vi "Clamp Max.vi"() -> ()   [LabVIEW 2014]
doc: "This example demonstrates the capabilities of the Max Clamp algorithm on a test image. You can also use this example to experiment using your own images and settings."
uses:
  <vilib>/vision/NI_Vision_Development_Module.lvlib
panel:
  in  "Clamp Settings":T1={"Angle Range (+/-)"=5.0, "Edge Polarity"={"Start"=0, "End"=0}} {"Edge Polarity"."End" items=["Any", "Rising", "Falling"]; "Edge Polarity"."Start" items=["Any", "Rising", "Falling"]}
  out "Clamp Results":T2 {"Angle (Relative)" format="%.3f"; "Angle (Absolute)" format="%.3f"; "Distance (Real World)" format="%.3f"; "Distance (Pixels)" format="%.3f"}
  in  "Curve Extraction Settings":T3={"Extraction Mode"=0, "Edge Threshold"=40, "Edge Filter Size"=1, "Min Length"=15, "Row Search Step Size"=10, "Col Search Step Size"=10, "Max Endpoint Gap"=5, "Closed"=FALSE, "Subpixel"=FALSE} {"Max Endpoint Gap" min=0; "Col Search Step Size" min=1 max=255 step=1; "Row Search Step Size" min=1 max=255 step=1; "Min Length" min=0; "Edge Filter Size" items=["Fine", "Normal", "Contour Tracing"]; "Edge Threshold" min=1 max=350 step=1; "Extraction Mode" items=["Normal", "Uniform Regions"]}
  out "Image":T4(plugin-control)
  in  "Stop":bool
  # "Overview: Demonstrates how to use the IMAQ Clamp Max function to find the maximum distance between the curves of an object.\nRequirements: Vision Development Software.\nInstructions:\n1. Run the VI.\n2. Draw a Region of Interest in the image or change the Curve Extraction Settings or Clamp Settings to see how the Max Clamp function works."
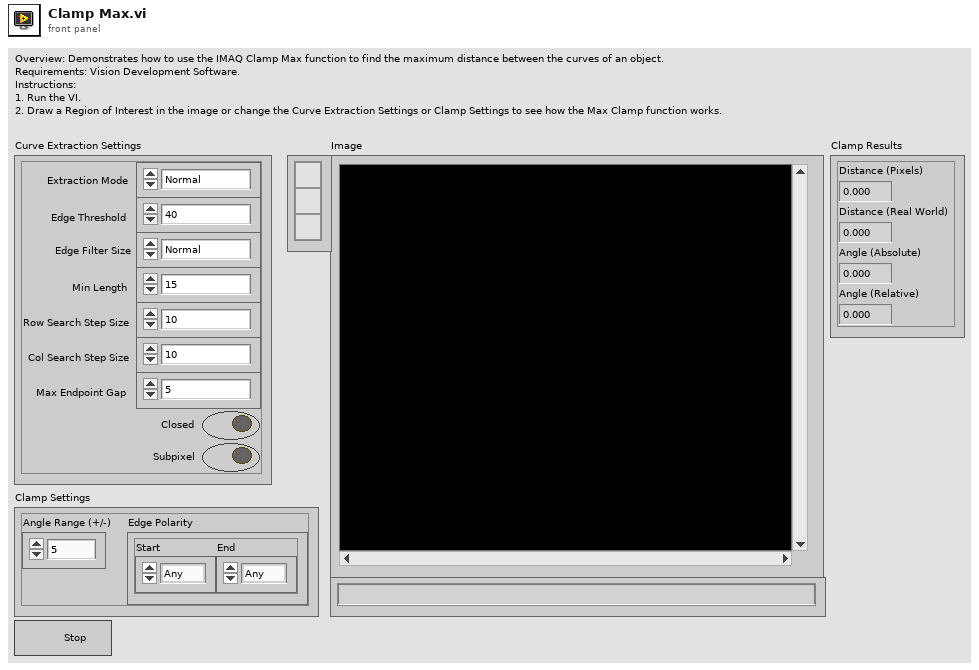
[diagram p1: front panel]
types:
  T1 = cluster{"Angle Range (+/-)":dbl, "Edge Polarity":cluster{"Start":u32, "End":u32}}
  T2 = cluster{"Distance (Pixels)":dbl, "Distance (Real World)":dbl, "Angle (Absolute)":dbl, "Angle (Relative)":dbl}
  T3 = cluster{"Extraction Mode":u32, "Edge Threshold":i32, "Edge Filter Size":u32, "Min Length":i32, "Row Search Step Size":i32, "Col Search Step Size":i32, "Max Endpoint Gap":i32, "Closed":bool, "Subpixel":bool}
  T4 = typedef "IMAQ Image.ctl" = refnum<image>
  T5 = typedef "ROI Descriptor" = cluster{"Global Rectangle":i32[], "Contours":cluster{"ID":enum32{"External", "Internal"}, "Type":u32, "Coordinates":i32[]}[]}
  T6 = typedef "Image Type" = u32
  T7 = cluster{"Show Search Area":bool, "Show Curves":bool, "Show Clamp Locations":bool, "Show Result":bool, "Search Area Color":u32, "Curves Color":u32, "Clamp Locations Color":u32, "Result Color":u32, "Overlay Group Name":string}
  T8 = cluster{"Global Rectangle":i32[], "Contours":cluster{"Contour Type":u32, "ROI Type":u32, "Points":i32[]}[]}
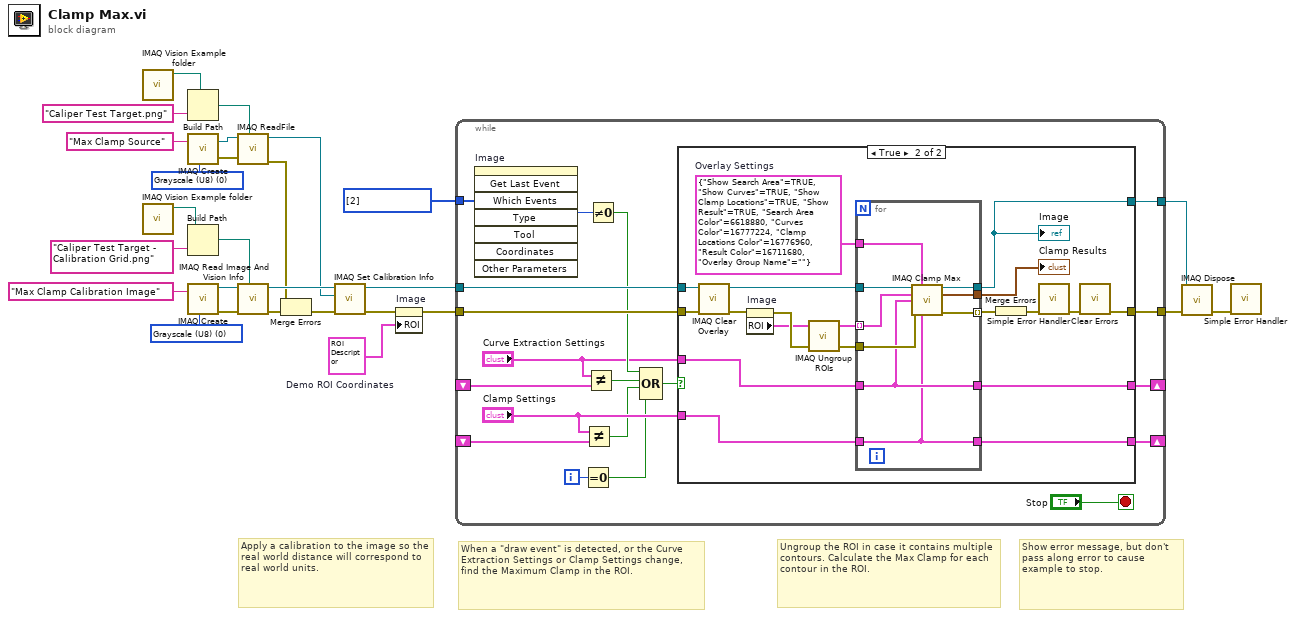
[diagram p0: block diagram]
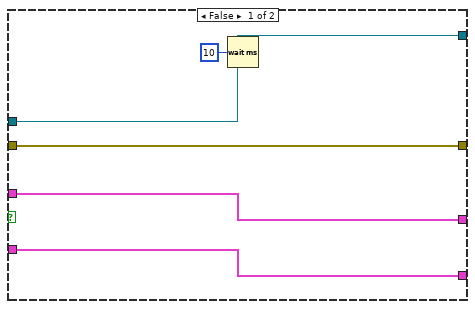
[diagram p2: hidden frame]
diagram:
  w8 = T5 {"Global Rectangle"=[94, 43, 1305, 1017], "Contours"=[{"ID"=enum."External", "Type"=12, "Coordinates"=[94, 214, 224, 312, 0]}, {"ID"=enum."External", "Type"=12, "Coordinates"=[232, 213, 372, 311, 321805]}, {"ID"=enum."External", "Type"=12, "Coordinates"=[143, 362, 220, 410, 0]}, {"ID"=enum."External", "Type"=12, "Coordinates"=[102, 475, 219, 529, 0]}, {"ID"=enum."External", "Type"=12, "Coordinates"=[226, 467, 369, 539, 315305]}, {"ID"=enum."External", "Type"=12, "Coordinates"=[221, 635, 380, 786, 359893]}, {"ID"=enum."External", "Type"=12, "Coordinates"=[538, 44, 687, 107, 359893]}, {"ID"=enum."External", "Type"=12, "Coordinates"=[501, 185, 671, 254, 359893]}, {"ID"=enum."External", "Type"=12, "Coordinates"=[501, 599, 671, 661, 359893]}, {"ID"=enum."External", "Type"=12, "Coordinates"=[729, 602, 899, 664, 314592]}, {"ID"=enum."External", "Type"=12, "Coordinates"=[491, 770, 679, 826, 0]}, {"ID"=enum."External", "Type"=12, "Coordinates"=[738, 781, 898, 817, 0]}, {"ID"=enum."External", "Type"=12, "Coordinates"=[498, 954, 669, 972, 0]}, {"ID"=enum."External", "Type"=12, "Coordinates"=[741, 949, 890, 974, 322432]}, {"ID"=enum."External", "Type"=12, "Coordinates"=[999, 450, 1293, 565, 0]}, {"ID"=enum."External", "Type"=12, "Coordinates"=[983, 106, 1305, 217, 0]}, {"ID"=enum."External", "Type"=12, "Coordinates"=[1152, 132, 1301, 191, 0]}, {"ID"=enum."External", "Type"=12, "Coordinates"=[961, 755, 1143, 952, 0]}, {"ID"=enum."External", "Type"=12, "Coordinates"=[233, 851, 379, 1005, 0]}]}  # Demo ROI Coordinates
  w12 = i32[] [2] items=["No Event"=0, "Click Event"=1, "Draw Event"=2, "Size Event"=4, "Scroll Event"=5, "Double Click Event"=8] ("Which Events")
  w26 = T6 0 items=["Grayscale (U8)", "Grayscale (I16)", "Grayscale (SGL)", "Complex (CSG)", "RGB (U32)", "HSL (U32)", "RGB (U64)", "Grayscale (U16)"] ("Image Type")
  w27 = T6 0 items=["Grayscale (U8)", "Grayscale (I16)", "Grayscale (SGL)", "Complex (CSG)", "RGB (U32)", "HSL (U32)", "RGB (U64)", "Grayscale (U16)"] ("Image Type")
  # "Show error message, but don't pass along error to cause example to stop."
  # "Ungroup the ROI in case it contains multiple contours. Calculate the Max Clamp for each contour in the ROI."
  # "When a \"draw event\" is detected, or the Curve Extraction Settings or Clamp Settings change, find the Maximum Clamp in the ROI."
  # "Apply a calibration to the image so the real world distance will correspond to real world units."
  n1 = call "IMAQ Vision Example folder.vi"() -> ("Example Image Path"=w16:path)  [unwired: 11 in]
  n2 = call "IMAQ Vision Example folder.vi"() -> ("Example Image Path"=w22:path)  [unwired: 11 in]
  n3 = Build Path(base path=w16, name or relative path="Caliper Test Target.png") -> (appended path=w15:path)
  n4 = call "IMAQ Create"("Image Name"="Max Clamp Source", "Image Type"=w27) -> ("New Image"=w18:T4, "error out"=w4:errorcluster)  [unwired: 2 in, 1 out]
  n5 = Build Path(base path=w22, name or relative path="Caliper Test Target - Calibration Grid.png") -> (appended path=w20:path)
  n6 = call "IMAQ Create"("Image Name"="Max Clamp Calibration Image", "Image Type"=w26) -> ("New Image"=w21:T4, "error out"=w5:errorcluster)  [unwired: 2 in, 1 out]
  n7 = call "IMAQ ReadFile"("File Path"=w15, "error in (no error)"=w4, "Image"=w18) -> ("error out"=w3:errorcluster, "Image Out"=w14:T4)  [unwired: 2 in, 5 out]
  n8 = call "IMAQ Read Image And Vision Info"("File Path"=w20, "error in (no error)"=w5, "Image"=w21) -> ("error out"=w2:errorcluster, "Image Out"=w19:T4)  [unwired: 1 in, 6 out]
  n9 = Merge Errors(w3, w2) -> (w1:errorcluster)
  n10 = call "IMAQ Set Calibration Info"("error in (no error)"=w1, "Image Dst"=w14, "Image Src"=w19) -> ("error out"=w7:errorcluster, "Calibrated Image"=w13:T4)  [unwired: 1 in, 6 out]
  n11 = property on="Image" class="ImageControl"(error in=w7, "ROI"=w8) -> (error out=w6:errorcluster)  [unwired: 1 in, 1 out]
  n12 = while {
    tunnel: w13 -> [w42]
    tunnel: w6 -> [w43]
    tunnel: w12 -> [w45]
    tunnel: [w29] -> w10
    tunnel: [w28] -> w11
    shift-right: [w31] -> _
    shift-left: _ -> [w41]
    shift-right: [w30] -> _
    shift-left: _ -> [w39]
    i -> [w46]
    stop <- "Stop" stop-if-true
    n13 = invoke on="Image" class="ImageControl" method="Get Last Event"("Which Events"=w45) -> ("Type"=w35:i32)  [unwired: 7 in, 7 out]
    n14 = Equal To 0?(x=w46) -> (x = 0?=w36:bool)
    n15 = Not Equal?(x="Clamp Settings", y=w41) -> (x != y?=w37:bool)
    n16 = Not Equal?(x="Curve Extraction Settings", y=w39) -> (x != y?=w38:bool)
    n17 = Not Equal To 0?(x=w35) -> (x != 0?=w34:bool)
    n18 = Compound Arithmetic op=OR(w34, w38, w37, w36) -> (w33:bool)
    n19 = case shown="True" w33 {
      tunnel: w42 -> [w47 w70]
      tunnel: w43 -> [w48 w69]
      tunnel: "Clamp Settings" -> [w50 w52]
      tunnel: "Curve Extraction Settings" -> [w49 w62]
      tunnel: [w50 w56] -> w31
      tunnel: [w49 w57] -> w30
      tunnel: [w48 w54] -> w29
      tunnel: [w47 w53] -> w28
      frame False {
        n20 = Wait (ms)(milliseconds to wait=u32 10) -> ()  [unwired: 1 out]
      }
      frame True {
        w61 = T7 {"Show Search Area"=TRUE, "Show Curves"=TRUE, "Show Clamp Locations"=TRUE, "Show Result"=TRUE, "Search Area Color"=6618880, "Curves Color"=16777224, "Clamp Locations Color"=16776960, "Result Color"=16711680, "Overlay Group Name"=""}  # Overlay Settings
        n21 = call "IMAQ Clear Overlay"("error in (no error)"=w69, "Image"=w70) -> ("error out"=w66:errorcluster, "Image Out"=w63:T4)  [unwired: 1 in, 7 out]
        n22 = property on="Image" class="ImageControl"(error in=w66) -> (error out=w68:errorcluster, "ROI"=w67:T8)  [unwired: 1 in, 1 out]
        n23 = call "IMAQ Ungroup ROIs"("error in (no error)"=w68, "ROI Descriptor"=w67) -> ("error out"=w64:errorcluster, "ROI Descriptors out"=w65:T5[])  [unwired: 2 in]
        n24 = for {
          tunnel: w63 -> [w79]
          tunnel: w65 -> [w78] mode=indexing
          tunnel: w64 -> [w77]
          tunnel: w62 -> [w72]
          tunnel: w52 -> [w71]
          tunnel: w61 -> [w76]
          tunnel: [w75] -> w53
          tunnel: [w74] -> w58
          tunnel: [w73] -> w60 mode=indexing
          tunnel: [w72] -> w57
          tunnel: [w71] -> w56
          n25 = call "IMAQ Clamp Max"("Source Image"=w79, "Overlay Settings"=w76, "ROI Descriptor"=w78, "Curve Extraction Settings"=w72, "error in (no error)"=w77, "Clamp Settings"=w71) -> ("Image Out"=w75:T4, "Clamp Results"=w74:T2, "error out"=w73:errorcluster)  [unwired: 1 in, 6 out]
        }
        "Clamp Results" <- w58
        "Image" <- w53
        n26 = Merge Errors(w60) -> (w59:errorcluster)
        n27 = call <vilib>:"Simple Error Handler.vi"("error in (no error)"=w59) -> ("error out"=w55:errorcluster)  [unwired: 4 in, 4 out]
        n28 = call <vilib>:"Clear Errors.vi"("error in (no error)"=w55) -> ("error out"=w54:errorcluster)  [unwired: 5 in, 1 out]
      }
    }
  }
  n29 = call "IMAQ Dispose"("Image"=w11, "error in (no error)"=w10) -> ("error out"=w9:errorcluster)  [unwired: 4 in]
  n30 = call <vilib>:"Simple Error Handler.vi"("error in (no error)"=w9) -> ()  [unwired: 4 in, 5 out]
